vi "Calculate Start Point by Rows and Cols.vi"(8 "错误输入":errorcluster, 9 "Size":cluster{"x":i16, "y":i16}={"x"=50, "y"=50} caption="Size(w,h)", 10 "Start Point":cluster{"x":i16, "y":i16} caption="Start (x,y)", 11 "Rows and Cols":i32[](array[numeric])) -> (0 "错误输出":errorcluster, 3 "Start Point Array":cluster{"x":i16, "y":i16}[](array[cluster]))   [LabVIEW 2011]
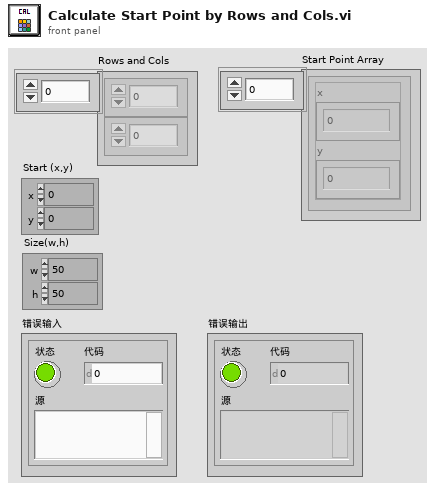
[diagram p1: front panel]
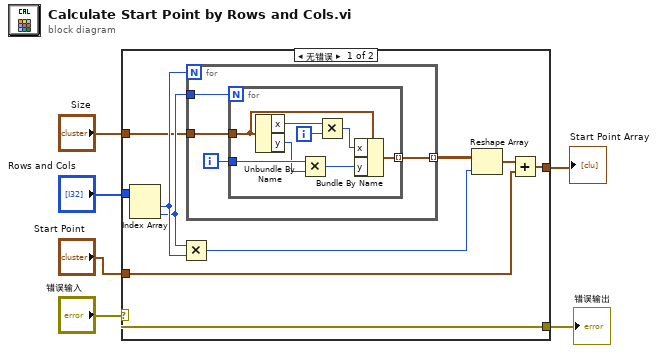
[diagram p0: block diagram]
diagram:
  n1 = case shown="无错误" "错误输入" {
    selector: "错误输入" -> [w11 w29]
    tunnel: [w11 w29] -> w5
    tunnel: "Size" -> [w10 _]
    tunnel: "Rows and Cols" -> [w9 _]
    tunnel: [w8 _] -> w2
    tunnel: "Start Point" -> [w7 _]
    frame No Error {
      n2 = Index Array(array=w9) -> (element #1=w15:i32, element #2=w12:i32)  [unwired: 2 in]
      n3 = Multiply(x=w12, y=w15) -> (x*y=w14:i32)
      n4 = for {
        N: w15 -> [_]
        tunnel: w12 -> [w20]
        tunnel: w10 -> [w18]
        tunnel: [w17] -> w16 mode=indexing
        i -> [w19]
        n5 = for {
          N: w20 -> [_]
          tunnel: w19 -> [w26]
          tunnel: w18 -> [w22]
          tunnel: [w21] -> w17 mode=indexing
          i -> [w27]
          n6 = Unbundle By Name(w22) -> ("x"=w28:i16, "y"=w25:i16)
          n7 = Multiply(x=w26, y=w25) -> (x*y=w23:i32)
          n8 = Multiply(x=w28, y=w27) -> (x*y=w24:i32)
          n9 = Bundle By Name(cluster=w22, "x"=w24, "y"=w23) -> (w21:cluster{"x":i16, "y":i16})
        }
      }
      n10 = Reshape Array(w16, w14) -> (w13:cluster{"x":i16, "y":i16}[])
      n11 = Add(x=w13, y=w7) -> (x+y=w8:cluster{"x":i16, "y":i16}[])
    }
    frame Error {
    }
  }
  "错误输出" <- w5
  "Start Point Array" <- w2
